vi "App - analyze RUS V6.vi"() -> ()   [LabVIEW 2015] (continued)
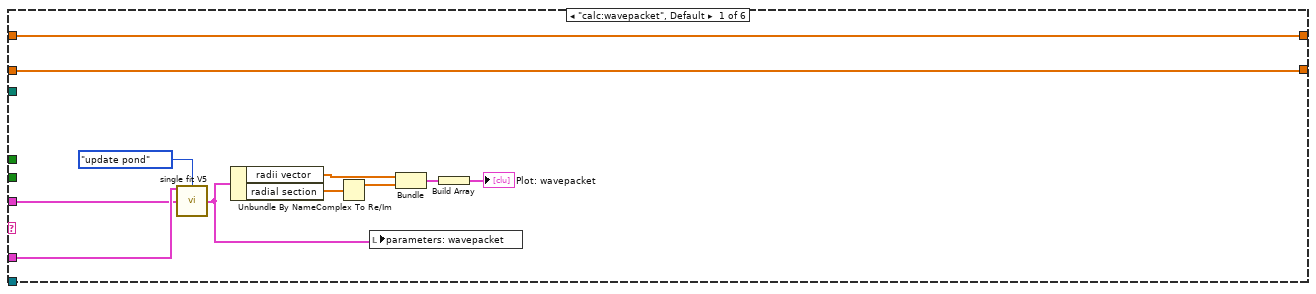
[diagram p2: hidden frame]
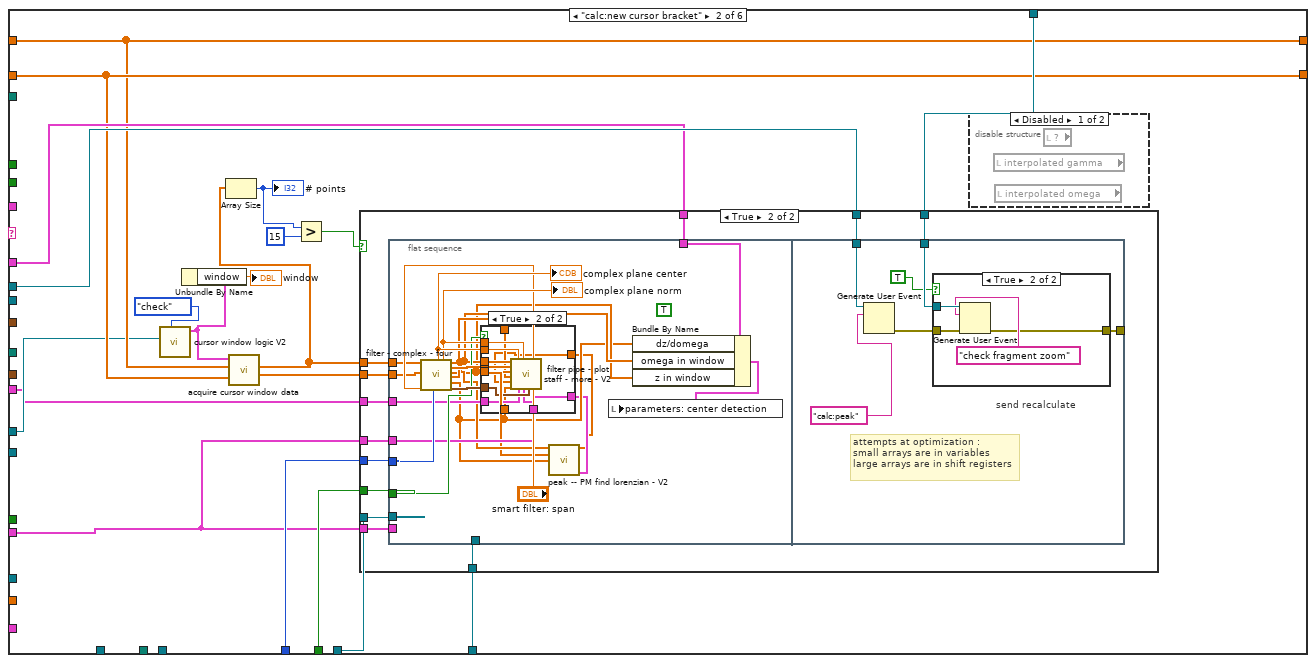
[diagram p3: hidden frame]
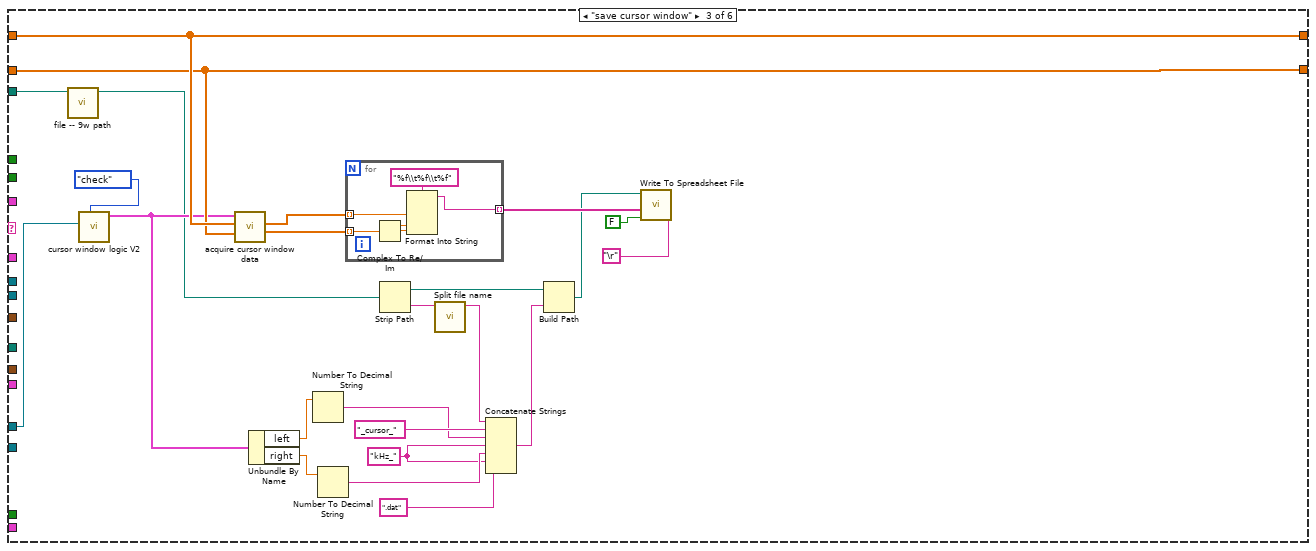
[diagram p8: hidden frame]
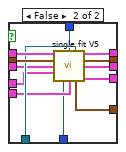
[diagram p9: hidden frame]
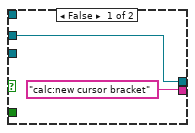
[diagram p10: hidden frame]
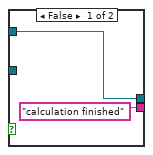
[diagram p11: hidden frame]
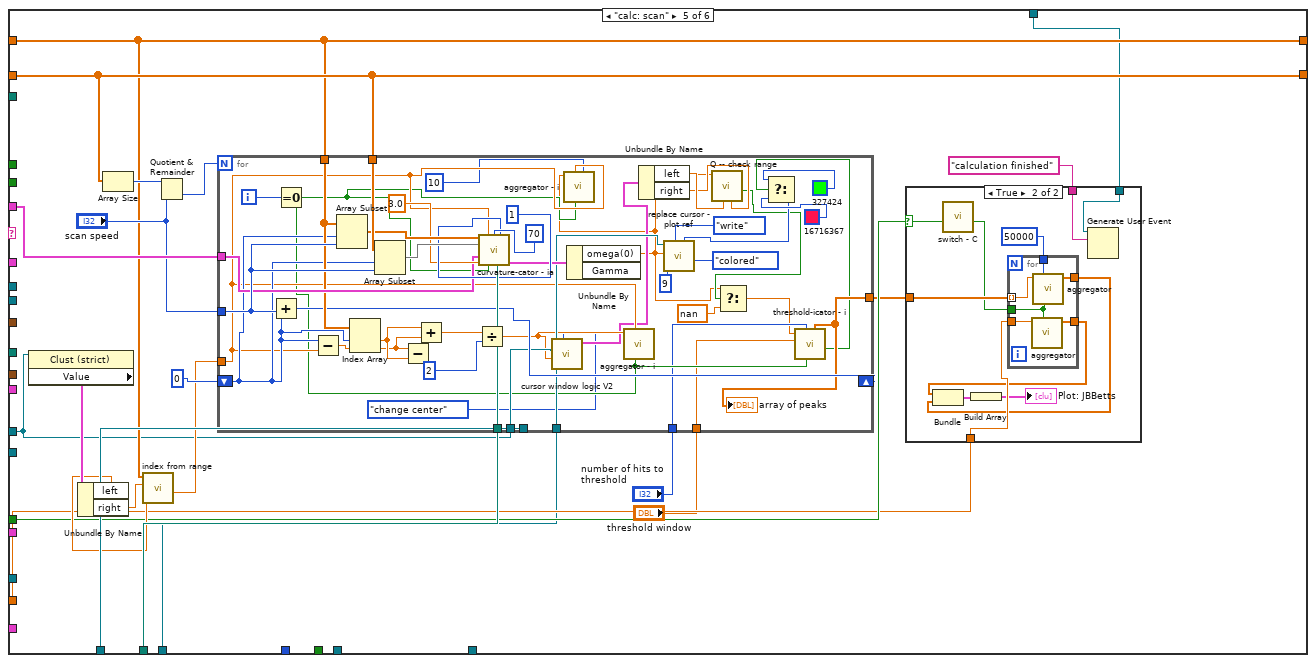
[diagram p12: hidden frame]
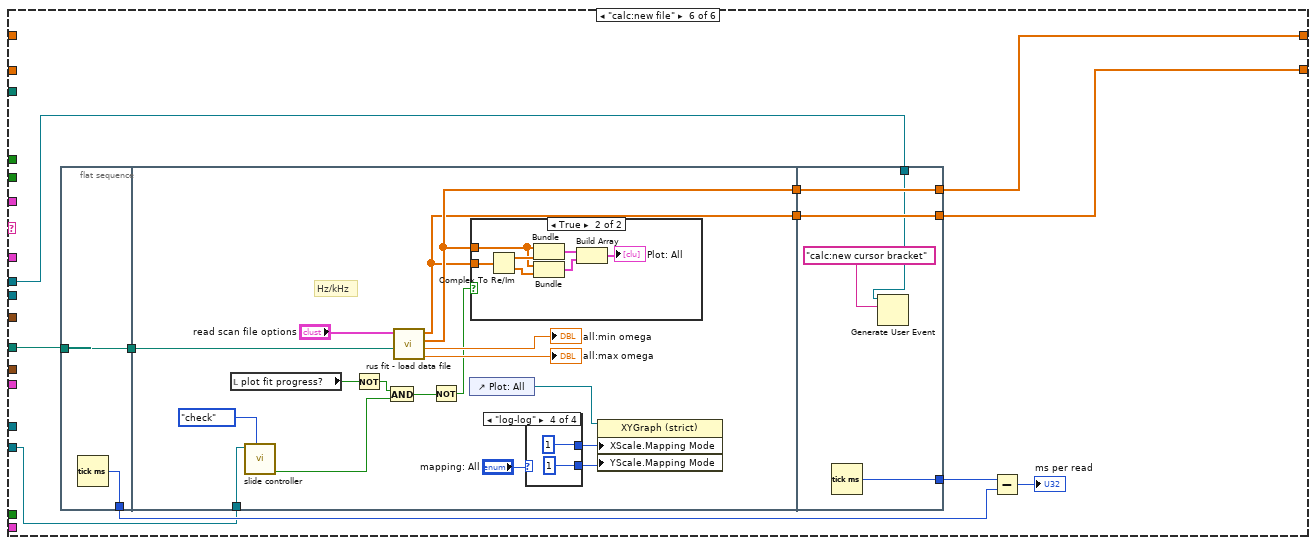
[diagram p14: hidden frame]
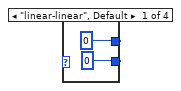
[diagram p15: hidden frame]
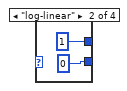
[diagram p16: hidden frame]
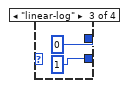
[diagram p17: hidden frame]
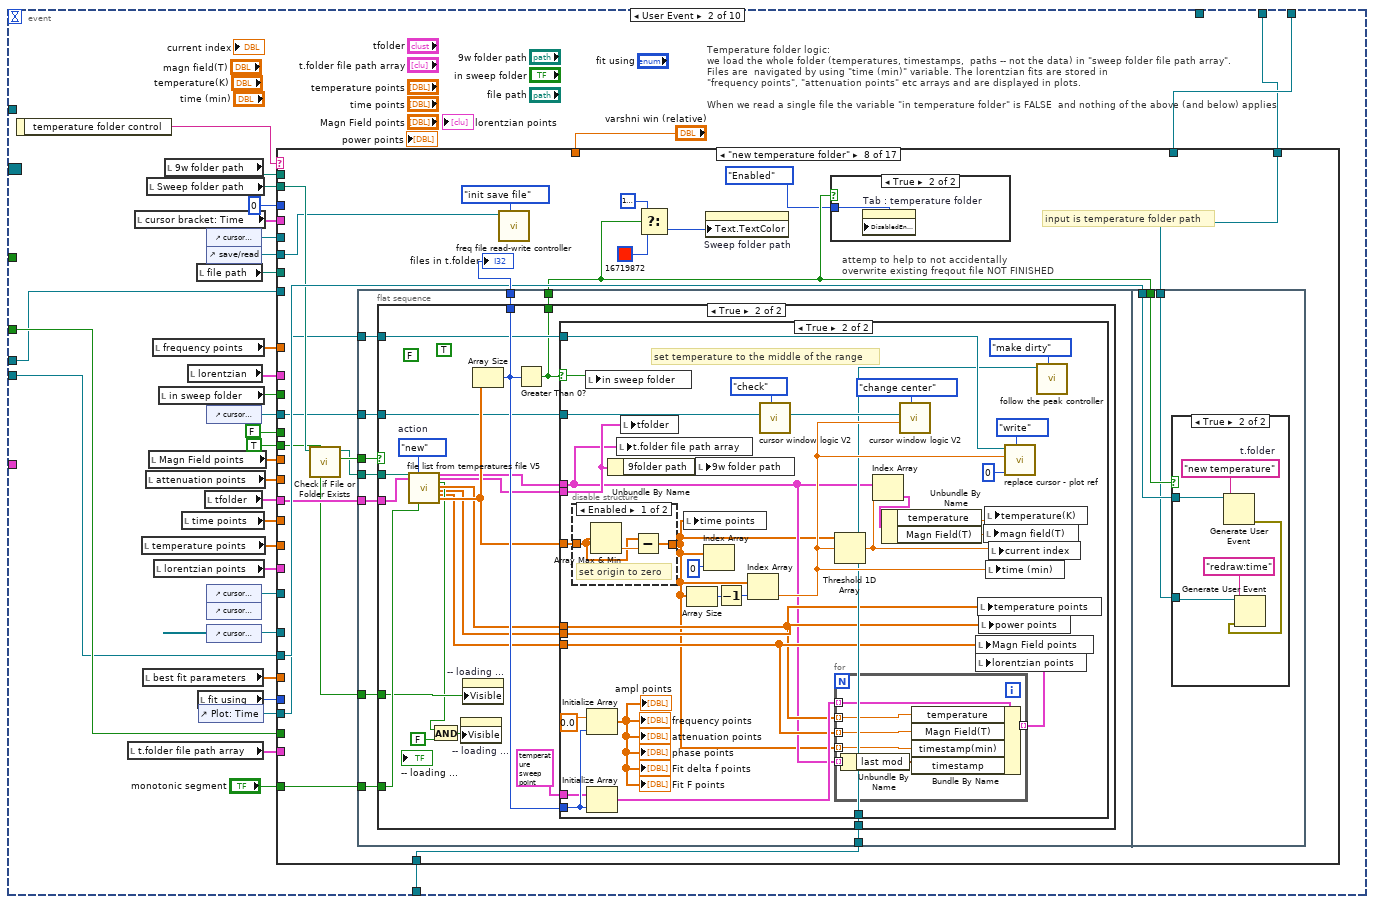
[diagram p19: hidden frame]
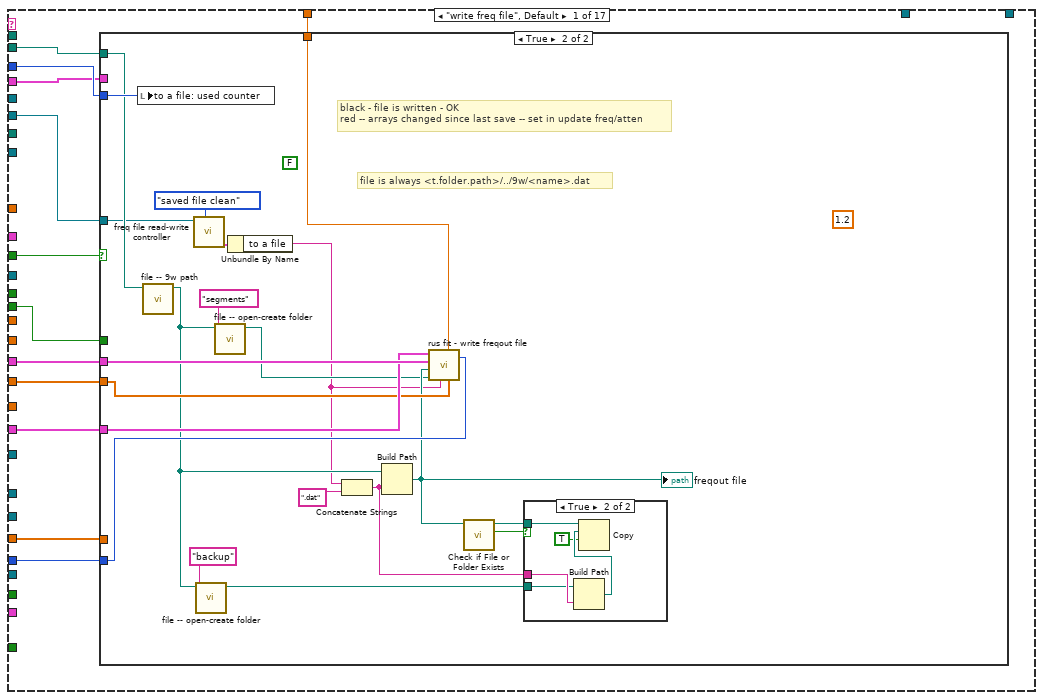
[diagram p20: hidden frame]
            w2168 = "lookup read from list"  # t.folder
            # "\"t\""
            n1015 = Generate User Event(user event=w2167, event data cluster=w2168) -> ()  [unwired: 2 in, 2 out]
          }
        }
      }
      event Mouse Down; Value Change {
        n1016 = event-data() -> ()  [unwired: 1 in, 1 out]
        n1017 = call "freq file read-write controller.vi"("action"=save-read_action."copy read from read ring", "save/read"=w2169) -> ()  [unwired: 7 in, 3 out]
      }
      event Mouse Down {
        # "if the text is not a number \nor it is a number but is outside the current frequency window \n\nthen \n\nset  name to a current  peak frequency -- if it exists"
        n1018 = event-data() -> ()  [unwired: 1 in, 1 out]
        n1019 = call "freq file read-write controller.vi"("action"=save-read_action."check", "save/read"=w2179) -> ("save read out"=w2181:T6)  [unwired: 7 in, 2 out]
        n1020 = Unbundle By Name(w2181) -> ("to a file"=w2180:string)
        n1021 = Unbundle By Name(w2183) -> ("left"=w2178:dbl, "right"=w2177:dbl)
        n1022 = Decimal String To Number(string=w2180) -> (offset past number=w2192:i32, number=w2176:i32)  [unwired: 2 in]
        n1023 = call "Q -- check range -- i -- real.vi"("upper"=w2177, "lower"=w2178, "number"=w2176) -> ("in range?"=w2172:bool)  [unwired: 6 in, 2 out]
        n1024 = Equal?(x=w2192, y=-1) -> (x = y?=w2190:bool)
        n1025 = Not(x=w2172) -> (.not. x?=w2171:bool)
        n1026 = Or(x=w2190, y=w2171) -> (x .or. y?=w2191:bool)
        n1027 = case shown="False" w2191 {
          selector: w2191 -> [w2199 _]
          tunnel: [w2200 TRUE] -> w2189
          frame False {
            n1028 = Not(x=w2199) -> (.not. x?=w2202:bool)
            n1029 = Less?(x="to a file: used counter", y=1) -> (x < y?=w2201:bool)
            n1030 = And(x=w2202, y=w2201) -> (x .and. y?=w2200:bool)
          }
          frame True {
          }
        }
        n1031 = Unbundle By Name(w2184) -> ("omega(0)"=w2174:dbl)
        n1032 = call "Q -- check range -- i -- real.vi"("lower"=0.0, "number"=w2174) -> ("in range?"=w2173:bool)  [unwired: 7 in, 2 out]
        n1033 = local read "to a file: used counter"() -> (w2186:i32)
        n1034 = Compound Arithmetic op=AND(w2173, w2189) -> (w2188:bool)
        n1035 = case shown="True" w2188 {
          tunnel: w2174 -> [_ w2195]
          tunnel: w2186 -> [w2193 w2198]
          tunnel: [w2193 w2197] -> w2185
          tunnel: w2179 -> [_ w2194]
          frame False {
          }
          frame True {
            n1036 = Increment(x=w2198) -> (x+1=w2197:i32)
            n1037 = call "freq file read-write controller.vi"("action"=save-read_action."set save file", "Numeric"=w2195, "save/read"=w2194) -> ()  [unwired: 6 in, 3 out]
          }
        }
        n1038 = local write "to a file: used counter"(w2185) -> ()
      }
      event "Plot: frequency vs T": Cursor Move {
        w2210 = enum16{"hide", "show x", "show y", "show (x,y)"}."show x"  # label
        (unwired) TRUE ("Boolean")
        w2218 = enum16{"", "read", "write"}."write"  # action
        w2207 = 0 ("index")
        w2206 = enum16{"", "read", "write"}."write" ("action")
        w2224 = enum16{"", "read", "write"}."read"  # action
        n1039 = event-data() -> ()  [unwired: 1 in, 4 out]
        n1040 = control-ref of="Plot: frequency vs T"() -> (w2213:refnum<vi>)
        n1041 = property on="Property Node" class="XYGraph (strict)"(reference=w2213) -> (reference out=w2211:refnum<vi>, "YScale.Maximum"=w2215:dbl, "YScale.Minimum"=w2214:dbl)  [unwired: 1 in, 1 out]
        n1042 = Add(x=w2215, y=w2214) -> (x+y=w2220:dbl)
        n1043 = Subtract(x=w2215, y=w2214) -> ()  [unwired: 1 out]
        n1044 = call "replace cursor - plot ref.vi"("action"=w2224, "cursor index"=0, "Plot ref in"=w2211) -> ("read X"=w2208:dbl, "Plot ref out"=w2212:refnum<vi>)  [unwired: 6 in, 1 out]
        n1045 = control-ref of="Plot: delta f"() -> (w2222:refnum<vi>)
        n1046 = control-ref of="Plot: attenuation vs T"() -> (w2221:refnum<vi>)
        n1047 = Divide(x=w2220, y=2.0) -> (x/y=w2216:dbl)
        n1048 = control-ref of="Plot: df/dT"() -> (w2209:refnum<vi>)
        n1049 = call "replace cursor - plot ref.vi"("label"=w2210, "action"=w2218, "cursor index"=0, "new  Y"=w2216, "Plot ref in"=w2212) -> ()  [unwired: 4 in, 3 out]
        n1050 = call "replace cursor - plot ref.vi"("action"=w2206, "cursor index"=w2207, "new X"=w2208, "Plot ref in"=w2222) -> ()  [unwired: 5 in, 3 out]
        n1051 = call "replace cursor - plot ref.vi"("action"=w2206, "cursor index"=w2207, "new X"=w2208, "Plot ref in"=w2221) -> ()  [unwired: 5 in, 3 out]
        n1052 = call "replace cursor - plot ref.vi"("action"=w2206, "cursor index"=w2207, "new X"=w2208, "Plot ref in"=w2209) -> ()  [unwired: 5 in, 3 out]
      }
      event "Plot: frequency vs T": Cursor Release {
        w2225 = enum16{"hide", "show x", "show y", "show (x,y)"}."hide"  # label
        w2226 = enum16{"", "read", "write"}."write"  # action
        w2227 = 0  # index
        n1053 = event-data() -> ()  [unwired: 1 in, 1 out]
        n1054 = control-ref of="Plot: frequency vs T"() -> (w2228:refnum<vi>)
        n1055 = call "replace cursor - plot ref.vi"("label"=w2225, "action"=w2226, "cursor index"=w2227, "Plot ref in"=w2228) -> ()  [unwired: 5 in, 3 out]
      }
      event "scale gauge: delta f plot": Value Change {
        n1056 = event-data() -> ()  [unwired: 1 in, 6 out]
        n1057 = local read "scale gauge: delta f plot"() -> (w2229:dbl)
        n1058 = local read "plot scale: delta f"() -> (w2231:T28)
        n1059 = call "control plot scale V1.vi"("action"=T41."manual zoom y", "fraction in"=w2229, "plot scale state"=w2231) -> ()  [unwired: 7 in, 2 out]
      }
      event "scale gauge: frequency vs T": Value Change {
        w2237 = 0.0  # t
        # "HACK!! fix this"
        n1060 = event-data() -> ()  [unwired: 1 in, 6 out]
        n1061 = local read "plot scale: frequency vs T"() -> (w2235:T28)
        n1062 = local read "scale gauge: frequency vs T"() -> (w2239:dbl)
        n1063 = Unbundle By Name(w2232) -> ("omega(0)"=w2236:dbl)
        n1064 = Not A Number/Path/Refnum?(number/path/refnum=w2236) -> (NaN/Path/Refnum?=w2238:bool)
        n1065 = Select(t=w2237, s=w2238, f=w2236) -> (s? t:f=w2234:dbl)
        n1066 = Bundle By Name(cluster=w2235, "center"=w2234) -> (w2233:T28)
        n1067 = call "control plot scale V1.vi"("action"=T41."manual zoom y", "fraction in"=w2239, "plot scale state"=w2233) -> ()  [unwired: 7 in, 2 out]
      }
      event "scale gauge: frequency vs H": Value Change {
        w2246 = 0.0  # t
        # "HACK!! fix this"
        n1068 = event-data() -> ()  [unwired: 1 in, 1 out]
        n1069 = local read "plot scale: frequency vs H"() -> (w2244:T28)
        n1070 = local read "scale gauge: frequency vs H"() -> (w2248:dbl)
        n1071 = Unbundle By Name(w2241) -> ("omega(0)"=w2245:dbl)
        n1072 = Not A Number/Path/Refnum?(number/path/refnum=w2245) -> (NaN/Path/Refnum?=w2247:bool)
        n1073 = Select(t=w2246, s=w2247, f=w2245) -> (s? t:f=w2243:dbl)
        n1074 = Bundle By Name(cluster=w2244, "center"=w2243) -> (w2242:T28)
        n1075 = call "control plot scale V1.vi"("action"=T41."manual zoom y", "fraction in"=w2248, "plot scale state"=w2242) -> ()  [unwired: 7 in, 2 out]
      }
      event Value Change {
        n1076 = event-data() -> ()  [unwired: 1 in, 6 out]
        n1077 = local read "scale gauge: All plot"() -> (w2252:T10)
        n1078 = Unbundle By Name(w2252) -> ("scale offset"=w2250:dbl, "scale range"=w2251:dbl)
        n1079 = local read "plot scale: All"() -> (w2253:T28)
        n1080 = call "control plot scale V1.vi"("offset in"=w2250, "action"=T41."manual zoom y", "fraction in"=w2251, "plot scale state"=w2253) -> ()  [unwired: 6 in, 2 out]
      }
      event Value Change {
        n1081 = event-data() -> ()  [unwired: 1 in, 6 out]
        n1082 = local read "scale gauge: Attenuation vs T"() -> (w2257:T10)
        n1083 = local read "plot scale: Attenuation vs T"() -> (w2258:T28)
        n1084 = Unbundle By Name(w2257) -> ("scale offset"=w2255:dbl, "scale range"=w2256:dbl)
        n1085 = call "control plot scale V1.vi"("offset in"=w2255, "action"=T41."manual zoom y", "fraction in"=w2256, "plot scale state"=w2258) -> ()  [unwired: 6 in, 2 out]
      }
      event Value Change {
        n1086 = event-data() -> ()  [unwired: 1 in, 1 out]
        n1087 = local read "scale gauge: Attenuation vs H"() -> (w2262:T10)
        n1088 = local read "plot scale: Attenuation vs H"() -> (w2263:T28)
        n1089 = Unbundle By Name(w2262) -> ("scale offset"=w2260:dbl, "scale range"=w2261:dbl)
        n1090 = call "control plot scale V1.vi"("offset in"=w2260, "action"=T41."manual zoom y", "fraction in"=w2261, "plot scale state"=w2263) -> ()  [unwired: 6 in, 2 out]
      }
      event "Plot: Time": Mouse Move {
        n1091 = event-data() -> ("Coords"=w2279:T55)  [unwired: 1 in]
        n1092 = disable-structure shown="Disabled" {
          frame Disabled {
            n1093 = control-ref of="Plot: frequency vs T"() -> (w2281:refnum<vi>)
            n1094 = invoke class="XYGraph (strict)" method="ObjHighlight"(reference=w2281) -> ()  [unwired: 2 in, 3 out]
            n1095 = property class="XYGraph (strict)"(reference=w2281) -> ("Plot"=w2280:refnum<vi>)  [unwired: 1 in, 2 out]
            n1096 = invoke class="XYGraph (strict)" method=#-1(reference=w2281) -> ()  [unwired: 2 in, 3 out]
            n1097 = property class="Plot" props=["Visible?"](reference=w2280) -> ()  [unwired: 1 in, 3 out]
            n1098 = invoke class="Plot" method="GetPlotAtPos"(reference=w2280) -> ()  [unwired: 4 in, 5 out]
          }
          frame Enabled {
          }
        }
        n1099 = invoke class="XYGraph (strict)" method="Map Coords To XY"(reference=w2269, "Coords"=w2279) -> ("XY"=w2278:cluster{"X":dbl, "Y":dbl})  [unwired: 5 in, 6 out]
        n1100 = local read "time points"() -> (w2272:dbl[])
        n1101 = local read "temperature points"() -> (w2267:dbl[])
        n1102 = Unbundle By Name(w2276) -> ("timestamp array"=w2277:dbl[])
        n1103 = Unbundle By Name(w2278) -> ("X"=w2273:dbl)
        n1104 = Threshold 1D Array(2:w2273, 3:w2272) -> (0:w2266:dbl)  [unwired: 1 in]
        n1105 = Index Array(array=w2267, index=w2266) -> (element=w2265:dbl)
        n1106 = Threshold 1D Array(2:w2273, 3:w2277) -> (0:w2275:dbl)  [unwired: 1 in]
        n1107 = Round Toward -Infinity(1:w2275) -> (0:→"section":dbl)
        n1108 = call "replace cursor - plot ref.vi"("action"=enum16{"", "read", "write"}."write", "cursor index"=1, "new X"=w2265, "Plot ref in"=w2268) -> ()  [unwired: 5 in, 3 out]
      }
      event "Plot: Time": Mouse Down {
        n1109 = event-data() -> ("Mods.Double Click"=w2285:bool)  [unwired: 1 in, 2 out]
        n1110 = case shown="True" w2285 {
          tunnel: w2287 -> [_ w2293]
          tunnel: w2286 -> [_ w2292]
          tunnel: w2284 -> [w2288 w2291]
          tunnel: [w2288 w2289] -> w2283
          frame False {
          }
          frame True {
            n1111 = flat-sequence {
              tunnel: w2293 -> [w2297]
              tunnel: w2292 -> [w2296]
              tunnel: ["redraw:freq/atten"] -> w2290
              frame #0 {
                n1112 = in-place {
                  in-place-border: w2296 -> [w2299]
                  n1113 = in-place-cluster #3(w2297) -> ("tfolder  -  file array"=w2300:T31[])
                  n1114 = in-place {
                    n1115 = in-place-array #4(w2300, w2299) -> (w2302:T31)
                    n1116 = in-place {
                      n1117 = in-place-cluster #5(w2302) -> ("active"=w2304:bool)
                      n1118 = Not(x=w2304) -> (.not. x?=w2303:bool)
                      n1119 = in-place-cluster #5("active"=w2303) -> (w2301:T31)
                    }
                    n1120 = in-place-array #4(w2301) -> (w2298:T31[])  [unwired: 1 out]
                  }
                  n1121 = in-place-cluster #3("tfolder  -  file array"=w2298) -> (w2295:T30)
                }
                n1122 = local write "tfolder"(w2295) -> ()
              }
            }
            n1123 = Generate User Event(user event=w2291, event data cluster=w2290) -> (user event out=w2289:refnum<user-event>)  [unwired: 2 in, 1 out]
          }
        }
        n1124 = Generate User Event(user event=w2283, event data cluster="redraw:time") -> ()  [unwired: 2 in, 2 out]
      }
      event "help (h)": Value Change {
        n1125 = event-data() -> ()  [unwired: 1 in, 1 out]
        n1126 = property on="help (h)" class="Bool" props=["Position"]() -> ()  [unwired: 2 in, 3 out]
        n1127 = Not(x="help toggle") -> (.not. x?=w2305:bool)
        n1128 = local write "help toggle"(w2305) -> ()
        n1129 = Control Help Window(1:w2305) -> ()  [unwired: 1 in]
      }
      event "scale gauge: df/dT plot": Value Change {
        n1130 = event-data() -> ()  [unwired: 1 in, 6 out]
        n1131 = local read "scale gauge: df/dT plot"() -> (w2309:dbl)
        n1132 = local read "plot scale: df/dT"() -> (w2308:T28)
        n1133 = call "control plot scale V1.vi"("action"=T41."manual zoom y", "fraction in"=w2309, "plot scale state"=w2308) -> ()  [unwired: 7 in, 2 out]
      }
      event "log-log": Value Change {
        n1134 = event-data() -> ("NewVal"=w2314:bool)  [unwired: 1 in, 1 out]
        n1135 = disable-structure shown="Disabled" {
          disable-tunnel: w2315 -> [w2323 _]
          disable-tunnel: w2314 -> [w2322 _]
          disable-tunnel: w2313 -> [w2320 _]
          disable-tunnel: w2312 -> [w2319 _]
          disable-tunnel: w2311 -> [w2318 _]
          frame Disabled {
            w2316 = u8 0  # Mapping Mode
            w2321 = u8 1  # Mapping Mode
            n1136 = Select(t=w2321, s=w2322, f=w2316) -> (s? t:f=w2317:u8)
            n1137 = property class="XYGraph (strict)"(reference=w2319, "YScale.Mapping Mode"=w2316, "XScale.Mapping Mode"=w2317) -> ()  [unwired: 1 in, 2 out]
            n1138 = property class="XYGraph (strict)"(reference=w2318, "YScale.Mapping Mode"=w2317, "XScale.Mapping Mode"=w2317) -> ()  [unwired: 1 in, 2 out]
            n1139 = property class="XYGraph (strict)"(reference=w2320, "YScale.Mapping Mode"=w2317, "XScale.Mapping Mode"=w2317) -> ()  [unwired: 1 in, 2 out]
            n1140 = property class="XYGraph (strict)"(reference=w2323, "YScale.Mapping Mode"=w2317, "XScale.Mapping Mode"=w2317) -> ()  [unwired: 1 in, 2 out]
          }
          frame Enabled {
          }
        }
      }
      event "Plot: frequency vs T": Mouse Down {
        w2328 = 0.0  # element
        n1141 = event-data() -> ()  [unwired: 1 in, 3 out]
        n1142 = local read "frequency points"() -> (w2329:dbl[])
        n1143 = Initialize Array(w2328, w2328) -> (w2327:dbl[])
        n1144 = local read "freq(T) : auto-adjust Y scale"() -> (w2331:bool)
        n1145 = for {
          tunnel: w2329 -> [w2333] mode=indexing
          shift-right: [w2332] -> w2326
          shift-left: w2327 -> [w2334]
          n1146 = call "Q - not nan and not zero.vi"("Numeric"=w2333) -> ("Boolean"=w2335:bool)  [unwired: 10 in]
          n1147 = case shown="False" w2335 {
            tunnel: w2334 -> [w2336 w2339]
            tunnel: w2333 -> [_ w2338]
            tunnel: [w2336 w2337] -> w2332
            frame False {
            }
            frame True {
              n1148 = Build Array (concatenate)(w2339, w2338) -> (w2337:dbl[])
            }
          }
        }
        n1149 = Array Max & Min(array=w2326) -> (max value=w2325:dbl, min value=w2324:dbl)  [unwired: 2 out]
        n1150 = case shown="False" w2331 {
          tunnel: w2330 -> [w2352 _]
          tunnel: w2325 -> [w2351 _]
          tunnel: w2324 -> [w2350 _]
          frame False {
            w2345 = 2.0  # y
            w2346 = 2.0  # y
            w2348 = 1.2  # y
            n1151 = Add(x=w2351, y=w2350) -> (x+y=w2347:dbl)
            n1152 = Subtract(x=w2351, y=w2350) -> (x-y=w2349:dbl)
            n1153 = Divide(x=w2347, y=w2346) -> (x/y=w2342:dbl)
            n1154 = Multiply(x=w2349, y=w2348) -> (x*y=w2344:dbl)
            n1155 = Divide(x=w2344, y=w2345) -> (x/y=w2341:dbl)
            n1156 = Subtract(x=w2342, y=w2341) -> (x-y=w2340:dbl)
            n1157 = Add(x=w2342, y=w2341) -> (x+y=w2343:dbl)
            n1158 = property on="Property Node" class="XYGraph (strict)"(reference=w2352, "YScale.Maximum"=w2343, "YScale.Minimum"=w2340) -> ()  [unwired: 1 in, 2 out]
          }
          frame True {
          }
        }
      }
      event "scale gauge: Plot: complex plane - filter": Value Change {
        n1159 = event-data() -> ("NewVal"=w2353:dbl)  [unwired: 1 in, 1 out]
        n1160 = local read "complex plane center"() -> (w2355:cdb)
        n1161 = control-ref of="Plot: complex plane - filter"() -> (w2354:refnum<vi>)
        n1162 = Complex To Re/Im(x + iy=w2355) -> (x=w2356:dbl, y=w2357:dbl)
        n1163 = Negate(x=w2353) -> (-x=w2362:dbl)
        n1164 = Add(x=w2357, y=w2362) -> (x+y=w2358:dbl)
        n1165 = Add(x=w2356, y=w2353) -> (x+y=w2360:dbl)
        n1166 = Add(x=w2356, y=w2362) -> (x+y=w2361:dbl)
        n1167 = Add(x=w2357, y=w2353) -> (x+y=w2359:dbl)
        n1168 = property on="Property Node" class="XYGraph (strict)"(reference=w2354, "XScale.Minimum"=w2361, "XScale.Maximum"=w2360, "YScale.Maximum"=w2359, "YScale.Minimum"=w2358) -> ()  [unwired: 1 in, 2 out]
      }
      event "plot filter progress?": Value Change {
        w2363 = "show fit progress"  # event data
        n1169 = event-data() -> ()  [unwired: 1 in, 1 out]
        n1170 = Generate User Event(user event=w2364, event data cluster=w2363) -> ()  [unwired: 2 in, 2 out]
      }
      event "fiter staff": Value Change {
        n1171 = event-data() -> ()  [unwired: 1 in, 2 out]
        n1172 = Generate User Event(user event=w2367, event data cluster="filter" ("event data")) -> ()  [unwired: 2 in, 2 out]
      }
      event Value Change {
        (unwired) FALSE
        # "wavepacket parameters\n have changed: wavepacket \nis in dirty state"
        n1173 = event-data() -> ()  [unwired: 1 in, 2 out]
        n1174 = local read "parameters: center detection"() -> (w2373:T21)
        n1175 = local read "parameters: wavepacket"() -> (w2371:T16)
        n1176 = Unbundle By Name(w2373) -> ("number of 2D grid points"=w2374:i32)
        n1177 = control-ref of="Plot: center detection"() -> (w2372:refnum<vi>)
        n1178 = flat-sequence {
          tunnel: w2371 -> [w2382]
          tunnel: w2369 -> [w2381]
          tunnel: w2372 -> [w2376]
          tunnel: w2374 -> [w2375]
          tunnel: w2370 -> [w2383]
          frame #0 {
            n1179 = Bundle By Name(cluster=w2382, "wavepacket is"=w2381) -> (w2380:T16)
            n1180 = Unbundle By Name(w2380) -> ("wave number"=w2378:dbl)
            n1181 = local write "parameters: wavepacket"(w2380) -> ()
            n1182 = call "replace cursor - plot ref.vi"("action"=enum16{"", "read", "write"}."write", "cursor index"=0, "new  Y"=w2378, "new X"=w2375, "Plot ref in"=w2376) -> ()  [unwired: 4 in, 3 out]
          }
          frame #1 {
            n1183 = Generate User Event(user event=w2383, event data cluster="calc:wavepacket" ("event data")) -> ()  [unwired: 2 in, 2 out]
          }
        }
      }
      event "Plot: center detection": Cursor Move {
        n1184 = event-data() -> ("CursIdx"=w2386:i32)  [unwired: 1 in, 3 out]
        n1185 = flat-sequence {
          tunnel: w2386 -> [w2388]
          tunnel: [w2412] -> _
          tunnel: w2385 -> [w2413]
          frame #0 {
            # "update two parameters from \nposition of the cursor"
            n1186 = local read "parameters: center detection"() -> (w2411:T21)
            n1187 = local read "parameters: wavepacket"() -> (w2409:T16)
            n1188 = control-ref of="Plot: center detection"() -> (w2407:refnum<vi>)
            n1189 = call "replace cursor - plot ref.vi"("action"=enum16{"", "read", "write"}."read", "cursor index"=w2388, "Plot ref in"=w2407) -> ("read Y"=w2392:dbl, "read X"=w2390:dbl, "Plot ref out"=w2387:refnum<vi>)  [unwired: 6 in]
            n1190 = call "replace cursor - plot ref.vi"("label"=enum16{"hide", "show x", "show y", "show (x,y)"}."show (x,y)", "action"=enum16{"", "read", "write"}."write", "cursor index"=w2388, "new  Y"=w2392, "new X"=w2390, "Plot ref in"=w2387) -> ("read Y"=w2391:dbl, "read X"=w2389:dbl)  [unwired: 3 in, 1 out]
            n1191 = call "Q -- check range -- i -- integer.vi"("upper"="# of 2D grid points: max", "lower"="# of 2D grid points: min", "default"=100 ("cursor index"), "number"=w2389) -> ("number in range"=w2397:i32)  [unwired: 5 in, 2 out]
            n1192 = Bundle By Name(cluster=w2411, "number of 2D grid points"=w2397) -> (w2410:T21)
            n1193 = Add(x="wave vector: max", y="wave vector: min") -> (x+y=w2402:dbl)
            n1194 = Divide(x=w2402, y=2.0) -> (x/y=w2403:dbl)
            n1195 = call "Q -- check range -- i -- real.vi"("upper"="wave vector: max", "lower"="wave vector: min", "default"=w2403, "number"=w2391) -> ("number in range"=w2400:dbl)  [unwired: 5 in, 2 out]
            n1196 = Bundle By Name(cluster=w2409, "wavepacket is"=FALSE, "wave number"=w2400) -> (w2408:T16)
            n1197 = local write "parameters: center detection"(w2410) -> ()
            n1198 = local write "parameters: wavepacket"(w2408) -> ()
          }
          frame #1 {
            n1199 = Generate User Event(user event=w2413, event data cluster="calc:wavepacket" ("event data")) -> (error out=w2412:errorcluster)  [unwired: 2 in, 1 out]
          }
        }
      }
      event "Plot: center detection": Cursor Release {
        (unwired) 0 ("cursor index")
        n1200 = event-data() -> ("CursIdx"=w2416:i32)  [unwired: 1 in, 3 out]
        n1201 = local read "parameters: center detection"() -> (w2418:T21)
        n1202 = local read "parameters: wavepacket"() -> (w2420:T16)
        n1203 = Unbundle By Name(w2418) -> ("number of 2D grid points"=w2419:i32)
        n1204 = control-ref of="Plot: center detection"() -> (w2426:refnum<vi>)
        n1205 = local read "# of 2D grid points: min"() -> (w2422:i32)
        n1206 = local read "# of 2D grid points: max"() -> (w2423:i32)
        n1207 = local read "wave vector: min"() -> (w2424:dbl)
        n1208 = local read "wave vector: max"() -> (w2425:dbl)
        n1209 = Unbundle By Name(w2420) -> ("wave number"=w2421:dbl)
        n1210 = call "replace cursor - plot ref.vi"("action"=enum16{"", "read", "write"}."write", "cursor index"=w2416, "new  Y"=w2421, "new X"=w2419, "Plot ref in"=w2426) -> ("Plot ref out"=w2427:refnum<vi>)  [unwired: 4 in, 2 out]
        n1211 = Generate User Event(user event=w2415, event data cluster="calc:peak" ("event data")) -> ()  [unwired: 2 in, 2 out]
        n1212 = property on="Property Node" class="XYGraph (strict)"(reference=w2427, "XScale.Minimum"=w2422, "XScale.Maximum"=w2423, "YScale.Minimum"=w2424, "YScale.Maximum"=w2425) -> ()  [unwired: 1 in, 2 out]
      }
    }
  }
  n1213 = flat-sequence {
    tunnel: [w2453] -> w28
    frame #0 {
      # "initialize scale controls"
      n1214 = control-ref of="Plot: All"() -> (w2449:refnum<vi>)
      n1215 = control-ref of="Plot: df/dT"() -> (w2443:refnum<vi>)
      n1216 = Bundle By Name(cluster="plot scale: All", "Plot Ref"=w2449, "center"=0.0, "delta"=0.1, "scale cursor index"=10) -> (w2448:T28)
      n1217 = Bundle By Name(cluster="plot scale: df/dT", "Plot Ref"=w2443, "center"=0.0, "delta"=60.0, "scale cursor index"=10) -> (w2441:T28)
      n1218 = local write "plot scale: df/dT"(w2441) -> ()
      n1219 = local write "plot scale: All"(w2448) -> ()
      n1220 = control-ref of="Plot: geometry"() -> (w2474:refnum<vi>)
      n1221 = control-ref of="Plot: delta f"() -> (w2466:refnum<vi>)
      n1222 = Bundle By Name(cluster="plot scale: Geometry", "Plot Ref"=w2474, "center"=0.0, "delta"=100.0, "scale cursor index"=10) -> (w2453:T28)
      n1223 = Bundle By Name(cluster="plot scale: delta f", "Plot Ref"=w2466, "center"=0.0, "delta"=60.0, "scale cursor index"=10) -> (w2464:T28)
      n1224 = local write "plot scale: Geometry"(w2453) -> ()
      n1225 = local write "plot scale: delta f"(w2464) -> ()
      n1226 = control-ref of="Plot: frequency vs T"() -> (w2454:refnum<vi>)
      n1227 = control-ref of="Plot: attenuation vs T"() -> (w2470:refnum<vi>)
      n1228 = Bundle By Name(cluster="plot scale: frequency vs T", "Plot Ref"=w2454, "center"=0.0, "delta"=100.0, "scale cursor index"=10) -> (w2457:T28)
      n1229 = Bundle By Name(cluster="plot scale: Attenuation vs T", "Plot Ref"=w2470, "center"=0.0, "delta"=50.0, "scale cursor index"=10) -> (w2471:T28)
      n1230 = local write "plot scale: Attenuation vs T"(w2471) -> ()
      n1231 = local write "plot scale: frequency vs T"(w2457) -> ()
      n1232 = control-ref of="Plot: frequency vs H"() -> (w2430:refnum<vi>)
      n1233 = control-ref of="Plot: attenuation vs H"() -> (w2429:refnum<vi>)
      n1234 = Bundle By Name(cluster="plot scale: frequency vs H", "Plot Ref"=w2430, "center"=0.0, "delta"=50.0, "scale cursor index"=10) -> (w2432:T28)
      n1235 = Bundle By Name(cluster="plot scale: Attenuation vs H", "Plot Ref"=w2429, "center"=0.0, "delta"=50.0, "scale cursor index"=10) -> (w2431:T28)
      n1236 = local write "plot scale: frequency vs H"(w2432) -> ()
      n1237 = local write "plot scale: Attenuation vs H"(w2431) -> ()
    }
  }
